vi "Check_lockin_stuff.vi"() -> ()   [LabVIEW 2015]
uses:
  <vilib>/Analysis/4window.llb/Kaiser-Bessel Window (DBL).vi
  <vilib>/Waveform/WDTOps.llb/WDT Get Waveform Time Array DBL.vi
  <vilib>/Analysis/NI_AALPro.lvlib
panel:
  in  "beta":dbl format="%0.2f"
  out "Phase":dbl[](graph)
  out "phase":dbl
  out "amp":dbl
  out "x/y 2":dbl
  out "x/y":dbl
  out "Waveform Data 3":waveform(dbl)[](graph)
  out "Waveform Data":waveform(dbl)(graph)
  in  "Stop Button":bool
  in  "milliseconds to wait":u32=1000
  out "error out":errorcluster
  in  "error in (no error)":errorcluster
  out "VISA Refnum out":refnum<visa-resource-name>
  in  "Channels":u16[](array[ring])=[0] items=["Channel 1", "Channel 2", "Channel 3", "Channel 4", "Math 1", "Math 2", "Math 3", "Math 4", "Reference 1", "Reference 2", "Reference 3", "Reference 4"]
  in  "VISA Refnum in":refnum<visa-resource-name>
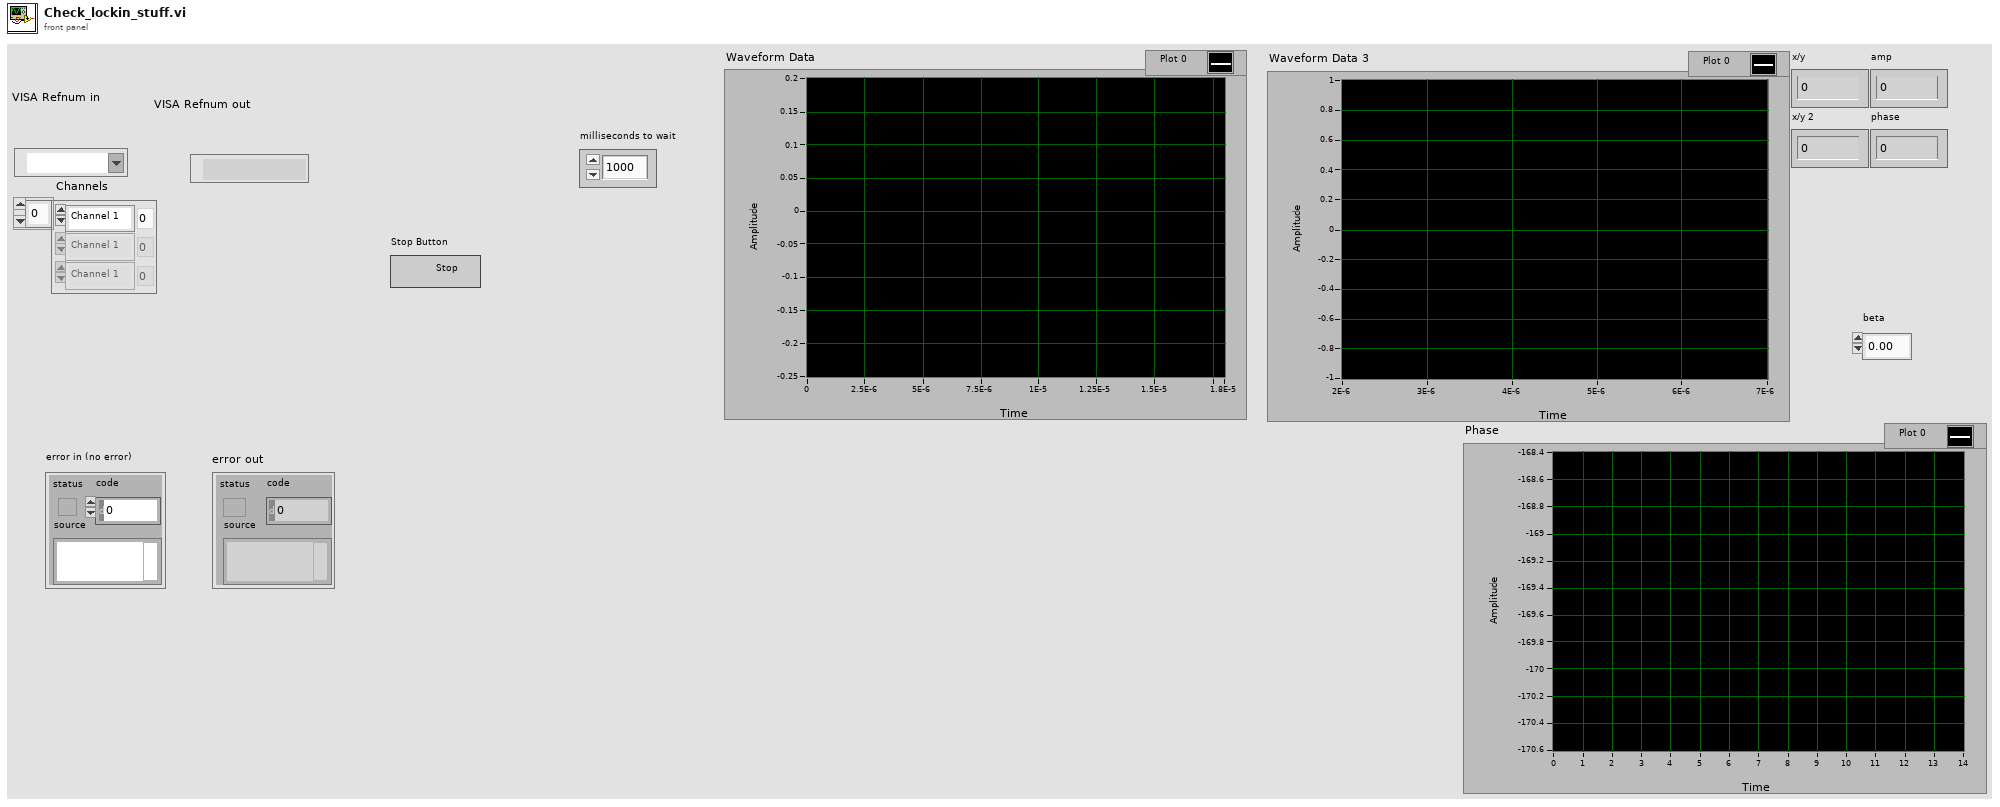
[diagram p1: front panel]
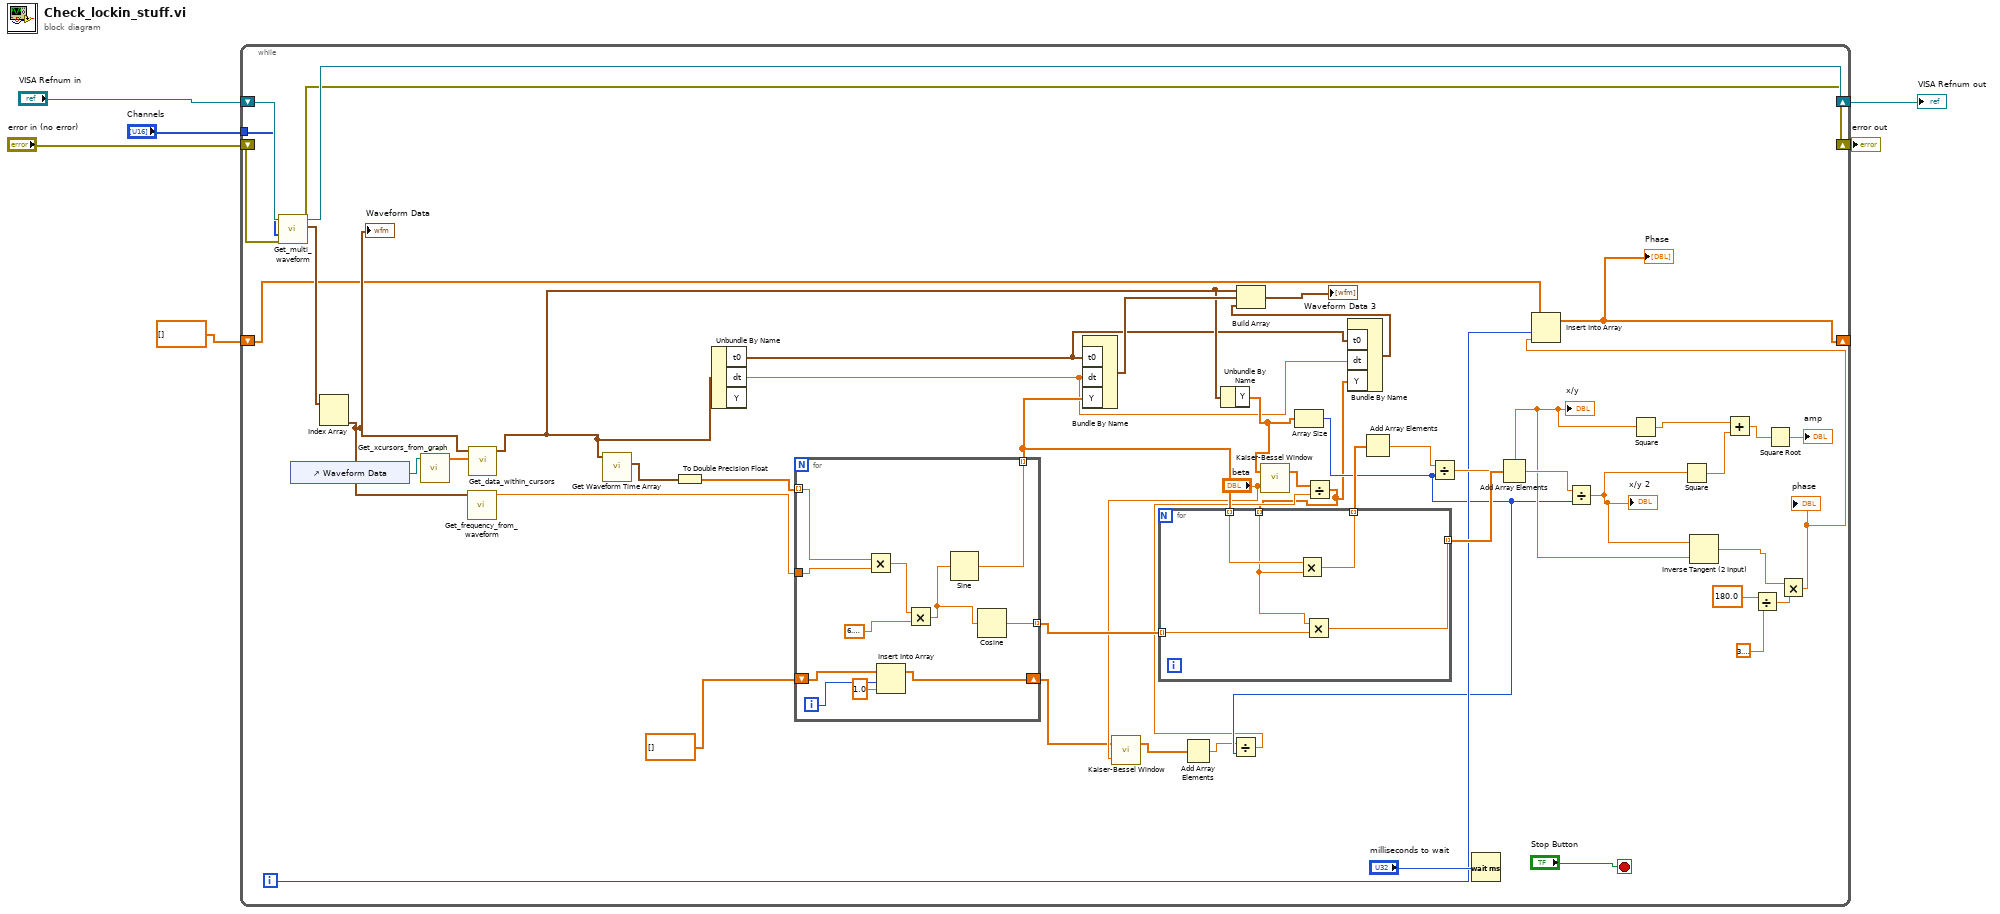
[diagram p0: block diagram]
diagram:
  n1 = while {
    tunnel: "Channels" -> [w55]
    shift-right: [w54] -> w4
    shift-left: "VISA Refnum in" -> [w56]
    shift-right: [w52] -> w2
    shift-left: "error in (no error)" -> [w53]
    shift-right: [w20] -> _
    shift-left: dbl[] [] -> [w22]
    i -> [w23]
    stop <- "Stop Button" stop-if-true
    n2 = call "Get_multi_waveform.vi"("error in (no error)"=w53, "Channels"=w55, "VISA Refnum in"=w56) -> ("error out"=w52:errorcluster, "Waveform Data"=w51:waveform(dbl)[], "VISA Refnum out"=w54:refnum<visa-resource-name>)  [unwired: 6 in]
    n3 = control-ref of="Waveform Data"() -> (w50:refnum<vi>)
    n4 = Index Array(array=w51) -> (element #2=w46:waveform(dbl))  [unwired: 2 in, 1 out]
    "Waveform Data" <- w46
    n5 = call "Get_xcursors_from_graph.vi"("WaveformGraph in"=w50) -> ("Array"=w49:dbl[])  [unwired: 10 in]
    n6 = call "Get_frequency_from_waveform.vi"("Waveform Data"=w46) -> ("Frequency"=w43:dbl)  [unwired: 9 in, 1 out]
    n7 = call "Get_data_within_cursors.vi"("Cursors"=w49, "Waveform Data"=w46) -> ("waveform out"=w39:waveform(dbl))  [unwired: 9 in]
    n8 = call-poly <vilib>:"Get Waveform Time Array.vi"("waveform in"=w39) -> ("X array"=w45:timestamp[])  [unwired: 9 in, 1 out]
    n9 = To Double Precision Float(number=w45) -> (double precision float=w44:dbl[])
    n10 = Unbundle By Name(w39) -> ("t0"=w8:timestamp, "dt"=w9:dbl)  [unwired: 1 out]
    n11 = for {
      tunnel: w44 -> [w72] mode=indexing
      tunnel: w43 -> [w71]
      tunnel: [w70] -> w40 mode=indexing
      tunnel: [w66] -> w36 mode=indexing
      shift-right: [w62] -> w16
      shift-left: dbl[] [] -> [w64]
      i -> [w65]
      n12 = Multiply(x=w72, y=w71) -> (x*y=w68:dbl)
      n13 = Insert Into Array(array=w64, index=w65, new element=1.0 ("new element/subarray")) -> (w62:dbl[])
      n14 = Multiply(x=w68, y=6.283185307179586) -> (x*y=w67:dbl)
      n15 = Sine(x=w67) -> (sin(x)=w70:dbl)
      n16 = Cosine(x=w67) -> (cos(x)=w66:dbl)
    }
    n17 = Bundle By Name("t0"=w8, "dt"=w9, "Y"=w40) -> (w42:waveform(dbl))  [unwired: 1 in]
    n18 = call-poly <vilib>:"Kaiser-Bessel Window.vi"("beta"="beta", "X"=w16) -> ("Windowed X"=w15:dbl[])  [unwired: 1 out]
    n19 = Add Array Elements(numeric array=w15) -> (sum=w13:dbl)
    n20 = Unbundle By Name(w39) -> ("Y"=w19:dbl[])
    n21 = call-poly <vilib>:"Kaiser-Bessel Window.vi"("beta"="beta", "X"=w19) -> ("Windowed X"=w12:dbl[])  [unwired: 1 out]
    n22 = Array Size(array=w19) -> (size(s)=w14:i32)
    n23 = Divide(x=w13, y=w14) -> (x/y=w11:dbl)
    n24 = Divide(x=w12, y=w11) -> (x/y=w10:dbl[])
    n25 = for {
      tunnel: w40 -> [w61] mode=indexing
      tunnel: w10 -> [w57] mode=indexing
      tunnel: [w60] -> w38 mode=indexing
      tunnel: w36 -> [w59] mode=indexing
      tunnel: [w58] -> w34 mode=indexing
      n26 = Multiply(x=w61, y=w57) -> (x*y=w60:dbl)
      n27 = Multiply(x=w57, y=w59) -> (x*y=w58:dbl)
    }
    n28 = Bundle By Name("t0"=w8, "dt"=w9, "Y"=w10) -> (w7:waveform(dbl))  [unwired: 1 in]
    n29 = Build Array(w39, w42, w7) -> (→"Waveform Data 3":waveform(dbl)[])
    n30 = Add Array Elements(numeric array=w38) -> (sum=w37:dbl)
    n31 = Divide(x=w37, y=w14) -> (x/y=w29:dbl)
    "x/y" <- w29
    n32 = Wait (ms)(milliseconds to wait="milliseconds to wait") -> ()  [unwired: 1 out]
    n33 = Add Array Elements(numeric array=w34) -> (sum=w35:dbl)
    n34 = Divide(x=w35, y=w14) -> (x/y=w28:dbl)
    "x/y 2" <- w28
    n35 = Square(x=w29) -> (x^2=w33:dbl)
    n36 = Square(x=w28) -> (x^2=w32:dbl)
    n37 = Inverse Tangent (2 Input)(1:w29, 2:w28) -> (0:w25:dbl)
    n38 = Add(x=w33, y=w32) -> (x+y=w31:dbl)
    n39 = Divide(x=180.0, y=3.141592653589793) -> (x/y=w24:dbl)
    n40 = Square Root(x=w31) -> (sqrt(x)=→"amp":dbl)
    n41 = Multiply(x=w25, y=w24) -> (x*y=w21:dbl)
    "phase" <- w21
    n42 = Insert Into Array(array=w22, index=w23, new element=w21) -> (w20:dbl[])
    "Phase" <- w20
  }
  "VISA Refnum out" <- w4
  "error out" <- w2
